vi "JBias.vi"(2 "C2":dbl, 3 "C1":dbl, 4 "T":dbl, 5 "t":dbl) -> (0 "f(t)":dbl, 1 "Jbias":dbl[](array[numeric]))   [LabVIEW 2021]
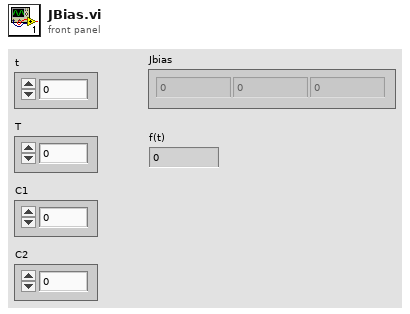
[diagram p1: front panel]
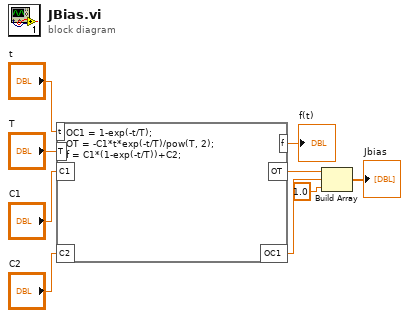
[diagram p0: block diagram]
diagram:
  n1 = formula code="OC1 = 1-exp(-t/T);\nOT = -C1*t*exp(-t/T)/pow(T, 2);\nf = C1*(1-exp(-t/T))+C2;"("t"="t", "T"="T", "C1"="C1", "C2"="C2") -> ("OT"=w8:dbl, "OC1"=w1:dbl, "f"=→"f(t)":dbl)
  n2 = Build Array(w8, w1, 1.0 ("element")) -> (→"Jbias":dbl[])
